vi "Prepare_Pulse_Seq.vi"() -> ()   [LabVIEW 2021]
uses:
  Drivers/Arduino_Pulse_Generator/Configurate/Channel_Pulse_Stream.ctl
  acefff95-97c1-4a03-be14-0b511ca0e7e1.vi
  db7f351c-eeeb-4ffc-aff2-0ba6d56ef54f.vi
  Pulse_Sequence_Global.vi
  <vilib>/Comparison/Less/Less Functor/Less Functor.lvclass
panel:
  in  "File Path":path=path "C:/Users/Daniel/Desktop/LabView/QST/Config_Files/channels_map_default.ini"
  out "Initial Array":T1[](array[typedef]) {"channel" min=2 max=13 step=1}
  in  "Reset All":bool
  in  "Reset Channel":bool
  out "Type of channel":string[](array[string])
  out "Times vs channel":dbl[][](array[numeric])
  in  "End configuration":bool
  in  "Stop":dbl
  in  "Start":dbl
  in  "Add Step":bool
  in  "Add Pulse":bool
  in  "Type of channel":u8(ring) items=["pump"=2, "probe"=3, "x pulse"=4, "y pulse"=5, "z pulse"=6, "z probe"=7]
  # "Note that units of time are not specified there.\nRemember that minimal pulse length is about 3,8 us."
  # "Add pulse with specific type\nbegining (start) and end (stop)"
  # "Add step with specific type\nand time (start)"
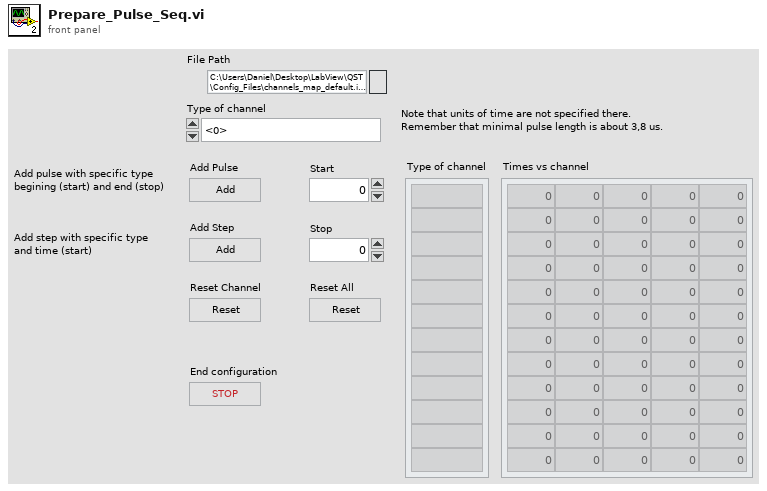
[diagram p1: front panel]
types:
  T1 = typedef "Channel_Pulse_Stream.ctl" = cluster{"Times":dbl[], "channel":u8}
  T2 = typedef "Channel_Cluster.ctl" = cluster{"Channel name":string, "Channel":u8}
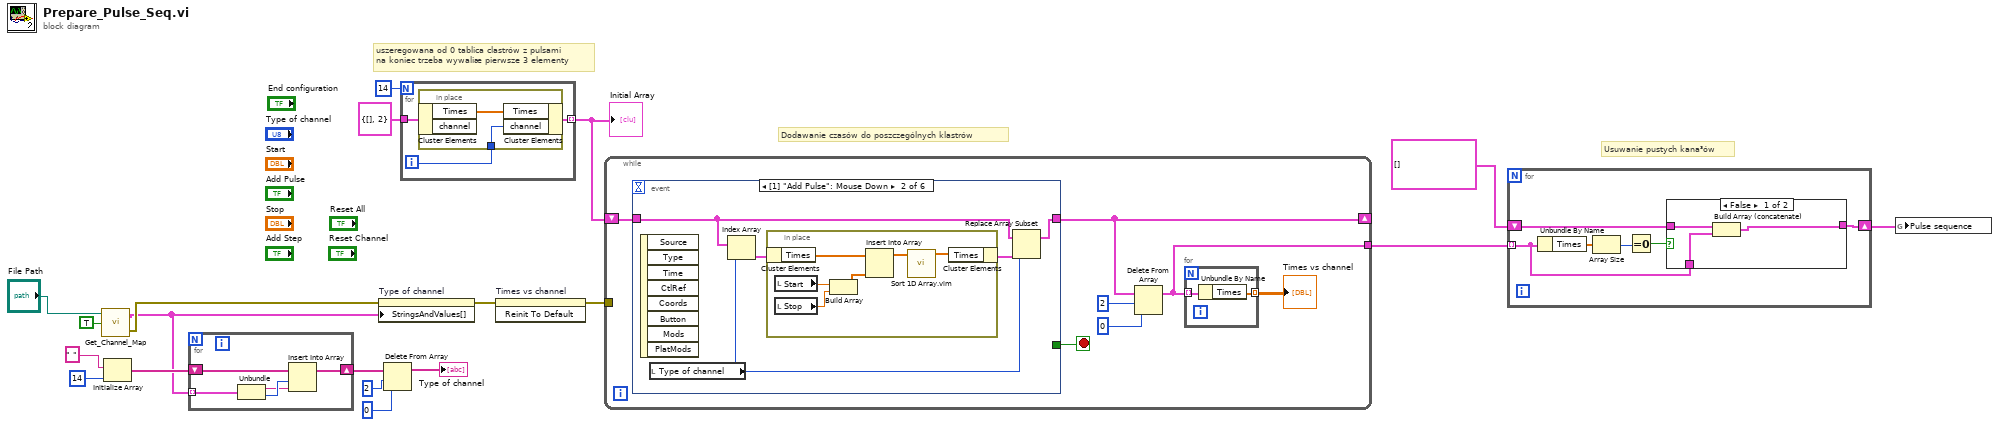
[diagram p0: block diagram]
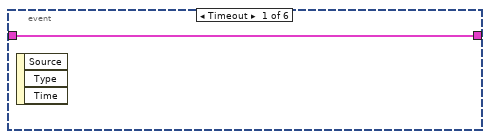
[diagram p3: hidden frame]
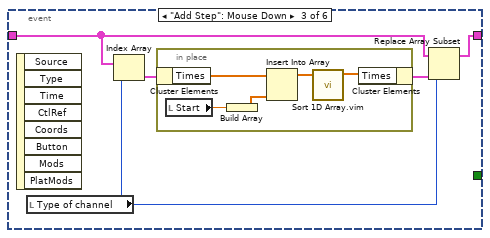
[diagram p4: hidden frame]
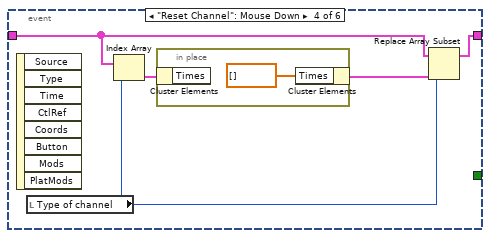
[diagram p5: hidden frame]
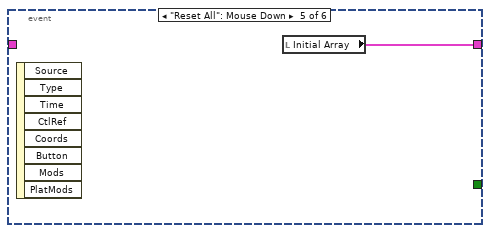
[diagram p6: hidden frame]
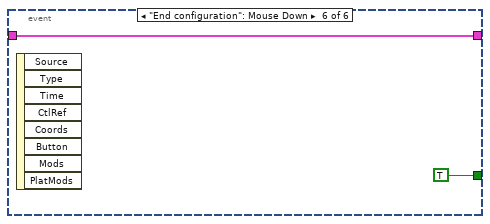
[diagram p7: hidden frame]
diagram:
  # "Usuwanie pustych kana³ów"
  # "uszeregowana od 0 tablica clastrów z pulsami\nna koniec trzeba wywaliæ pierwsze 3 elementy"
  # "Dodawanie czasów do poszczególnych klastrów"
  n1 = call "Get_Channel_Map.vi"("Get default(?)"=TRUE, "File Path"="File Path") -> ("error out"=w2:errorcluster, "Channels map"=w1:T2[])  [unwired: 1 in]
  n2 = Initialize Array(" ", 14 ("dimension size")) -> (w12:string[])
  n3 = for {
    tunnel: w1 -> [w22] mode=indexing
    shift-right: [w21] -> w11
    shift-left: w12 -> [w24]
    n4 = Unbundle(w22) -> ("Channel name"=w20:string, "Channel"=w23:u8)
    n5 = Insert Into Array(array=w24, index=w23, new element=w20) -> (w21:string[])
  }
  n6 = property on="Type of channel" class="Ring (strict)"(error in=w2, "StringsAndValues[]"=w1) -> (error out=w16:errorcluster)  [unwired: 1 in, 1 out]
  n7 = Delete From Array(array=w11, length=2, index=0) -> (array with subset deleted=→"Type of channel":string[])  [unwired: 1 out]
  n8 = for {
    N: 14 -> [_]
    tunnel: T1 {"Times"=[], "channel"=2} ("Channel pulse stream") -> [w27]
    tunnel: [w26] -> w17 mode=indexing
    i -> [w25]
    n9 = in-place {
      in-place-border: w25 -> [w29]
      n10 = in-place-cluster #1(w27) -> ("Times"=w28:dbl[])  [unwired: 1 out]
      n11 = in-place-cluster #1("Times"=w28, "channel"=w29) -> (w26:T1)
    }
  }
  "Initial Array" <- w17
  n12 = invoke on="Times vs channel" class="Arr (strict)" method="Reinit To Default"(error in=w16) -> (error out=w15:errorcluster)  [unwired: 2 in, 2 out]
  n13 = while {
    shift-right: [w32] -> _
    shift-left: w17 -> [w36]
    tunnel: [w30] -> w7
    tunnel: w15 -> [_]
    stop <- w35 stop-if-true
    n14 = event shown="[1] \"Add Pulse\": Mouse Down" {
      selector: _ -> [_ _ _ _ _ _]
      dyn-events: _ -> [_ _ _ _ _ _]
      timeout: _ -> [_ _ _ _ _ _]
      tunnel: w36 -> [w39 w42 w53 w63 _ w69]
      tunnel: [w39 w40 w51 w61 w67 w69] -> w32
      tunnel: [_ _ _ _ _ TRUE] -> w35
      event Timeout {
        n15 = event-data() -> ()  [unwired: 1 in, 3 out]
      }
      event "Add Pulse": Mouse Down {
        n16 = event-data() -> ()  [unwired: 1 in, 8 out]
        n17 = local read "Type of channel"() -> (w41:u8)
        n18 = Index Array(array=w42, index=w41) -> (element=w44:T1)
        n19 = in-place {
          n20 = in-place-cluster #2(w44) -> ("Times"=w48:dbl[])
          n21 = local read "Start"() -> (w49:dbl)
          n22 = local read "Stop"() -> (w50:dbl)
          n23 = Build Array(w49, w50) -> (w47:dbl[])
          n24 = Insert Into Array(array=w48, new element=w47) -> (w46:dbl[])  [unwired: 1 in]
          n25 = call "Sort 1D Array.vim"("unsorted array"=w46) -> ("sorted array"=w45:dbl[])  [unwired: 10 in]
          n26 = in-place-cluster #2("Times"=w45) -> (w43:T1)
        }
        n27 = Replace Array Subset(array=w42, new element=w43, index=w41) -> (w40:T1[])
      }
      event "Add Step": Mouse Down {
        n28 = event-data() -> ()  [unwired: 1 in, 8 out]
        n29 = local read "Type of channel"() -> (w52:u8)
        n30 = Index Array(array=w53, index=w52) -> (element=w55:T1)
        n31 = in-place {
          n32 = in-place-cluster #3(w55) -> ("Times"=w59:dbl[])
          n33 = local read "Start"() -> (w60:dbl)
          n34 = Build Array(w60) -> (w58:dbl[])
          n35 = Insert Into Array(array=w59, new element=w58) -> (w57:dbl[])  [unwired: 1 in]
          n36 = call "Sort 1D Array.vim"("unsorted array"=w57) -> ("sorted array"=w56:dbl[])  [unwired: 10 in]
          n37 = in-place-cluster #3("Times"=w56) -> (w54:T1)
        }
        n38 = Replace Array Subset(array=w53, new element=w54, index=w52) -> (w51:T1[])
      }
      event "Reset Channel": Mouse Down {
        n39 = event-data() -> ()  [unwired: 1 in, 8 out]
        n40 = local read "Type of channel"() -> (w62:u8)
        n41 = Index Array(array=w63, index=w62) -> (element=w65:T1)
        n42 = in-place {
          n43 = in-place-cluster #4(w65) -> ()  [unwired: 1 out]
          n44 = in-place-cluster #4("Times"=dbl[] []) -> (w64:T1)
        }
        n45 = Replace Array Subset(array=w63, new element=w64, index=w62) -> (w61:T1[])
      }
      event "Reset All": Mouse Down {
        n46 = event-data() -> ()  [unwired: 1 in, 8 out]
        n47 = local read "Initial Array"() -> (w67:T1[])
      }
      event "End configuration": Mouse Down {
        n48 = event-data() -> ()  [unwired: 1 in, 8 out]
      }
    }
    n49 = Delete From Array(array=w32, length=2, index=0) -> (array with subset deleted=w30:T1[])  [unwired: 1 out]
    n50 = for {
      tunnel: w30 -> [w38] mode=indexing
      tunnel: [w37] -> w31 mode=indexing
      n51 = Unbundle By Name(w38) -> ("Times"=w37:dbl[])
    }
    "Times vs channel" <- w31
  }
  n52 = for {
    shift-right: [w72] -> w5
    shift-left: T1[] [] -> [w71]
    tunnel: w7 -> [w70] mode=indexing
    n53 = Unbundle By Name(w70) -> ("Times"=w75:dbl[])
    n54 = Array Size(array=w75) -> (size(s)=w74:i32)
    n55 = Equal To 0?(x=w74) -> (x = 0?=w73:bool)
    n56 = case shown="False" w73 {
      tunnel: w71 -> [w78 w79]
      tunnel: [w76 w79] -> w72
      tunnel: w70 -> [w77 _]
      frame False {
        n57 = Build Array (concatenate)(w78, w77) -> (w76:T1[])
      }
      frame True {
      }
    }
  }
  n58 = global write "Pulse_Sequence_Global.vi" "Pulse sequence"(w5) -> ()
